vi "Reset Lock state.vi"(8 "error in (no error)":errorcluster, 9 "Boiler Simulation Controls":T1 {"Flame Sensor Value (%)" min=0.0 max=100.0 scale=0.0..100.0}, 10 "Indicator states in":T3 {"Time Count" format="%.2g"}, 11 "Runtime statuses in":T2) -> (0 "error out":errorcluster, 2 "Indicator states out":T3 {"Time Count" format="%.2g"}, 3 "Runtime statuses out":T2)   [LabVIEW 2014]
doc: "Checks runtime statuses and Control values. If Run Interlock is closed logs Boiler ready event and alows next state: Pre-Purge"
uses:
  Controls/Boiler Status Indicators.ctl
  Controls/Boiler runtime status indicators.ctl
  Controls/Boiler Simulation Controls.ctl
  Controls/Log file FGV action enum.ctl
  Controls/Log event enum.ctl
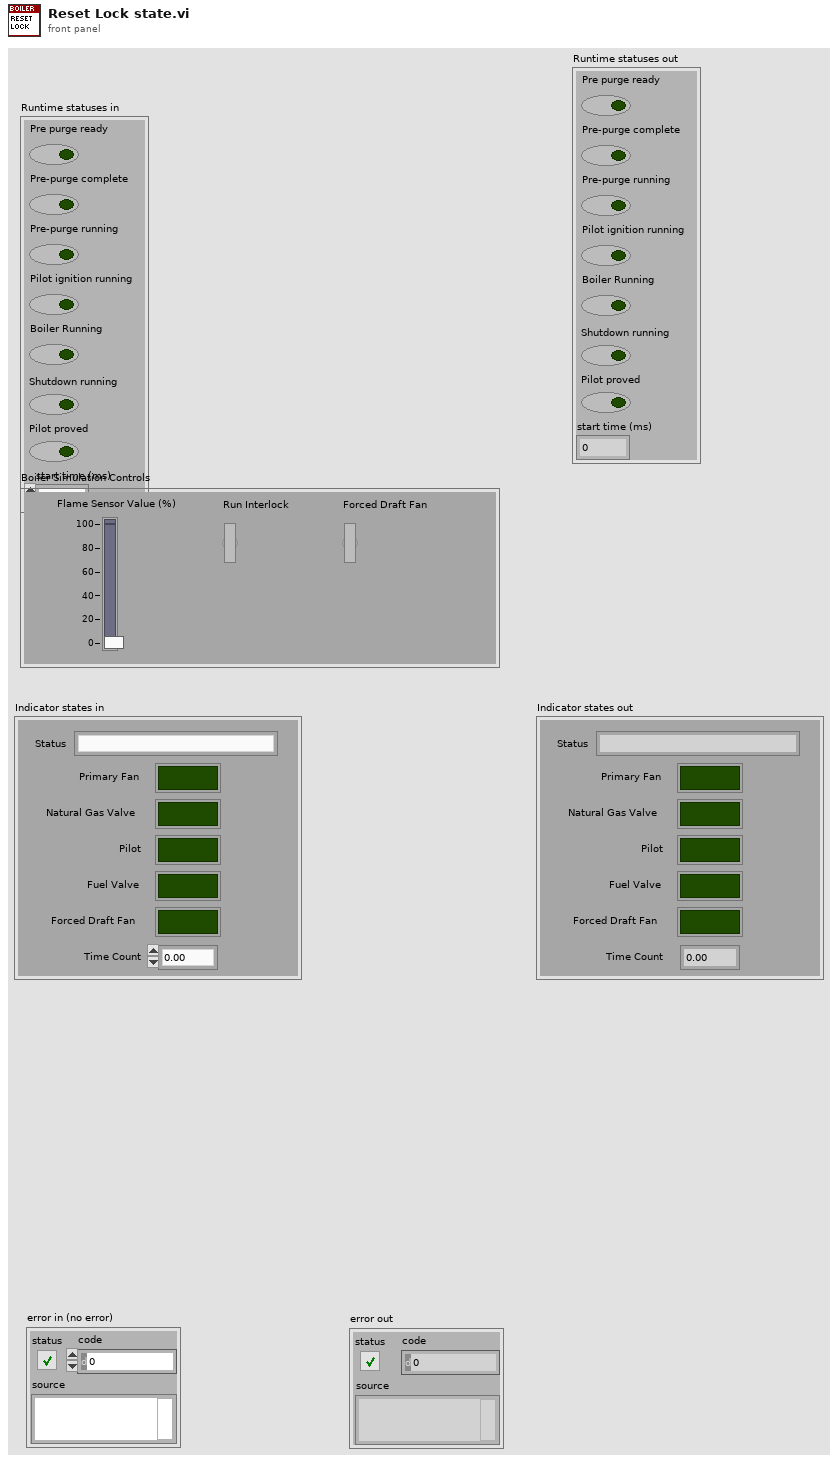
[diagram p1: front panel]
types:
  T1 = typedef "Boiler Simulation Controls.ctl" = cluster{"Flame Sensor Value (%)":dbl, "Run Interlock":bool, "Forced Draft Fan":bool}
  T2 = typedef "Boiler runtime status indicators.ctl" = cluster{"Pre purge ready":bool, "Pre-purge complete":bool, "Pre-purge running":bool, "Pilot ignition running":bool, "Boiler Running":bool, "Shutdown running":bool, "Pilot proved":bool, "start time (ms)":u32}
  T3 = typedef "Boiler Status Indicators.ctl" = cluster{"Status":string, "Primary Fan":bool, "Natural Gas Valve":bool, "Pilot":bool, "Fuel Valve":bool, "Forced Draft Fan":bool, "Time Count":dbl}
  T4 = typedef "Log event enum.ctl" = enum16{"Boiler Initialized", "Boiler Ready", "Start Pre-Purge", "Pre-Purge Complete", "Pilot ON", "Pilot proved", "Forced Draft Fan ON", "Boiler Running", "Start Shutdown Purge", "Shutdown Purge Complete"}
  T5 = typedef "Log file FGV action enum.ctl" = enum16{"open log file", "log event", "close log file"}
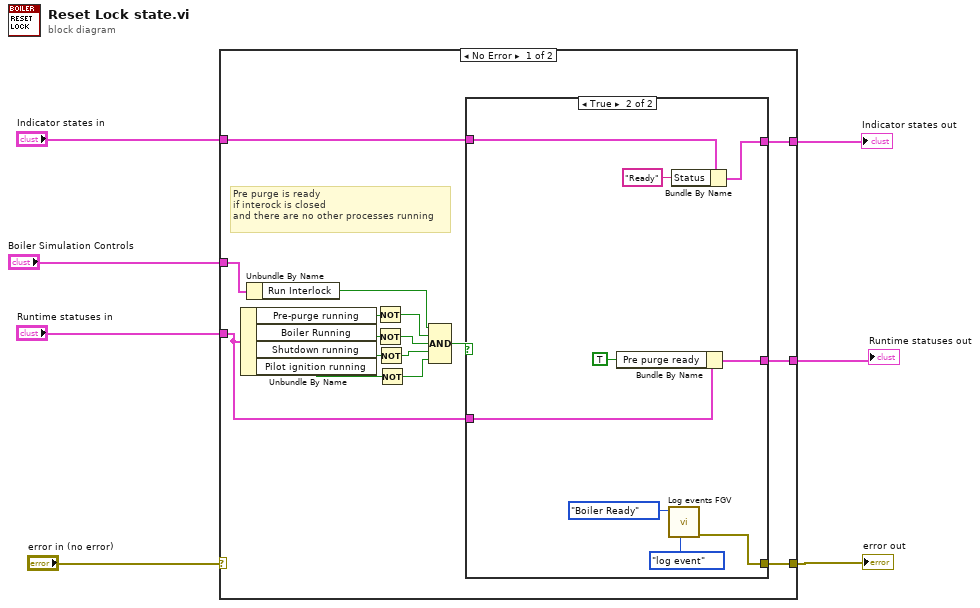
[diagram p0: block diagram]
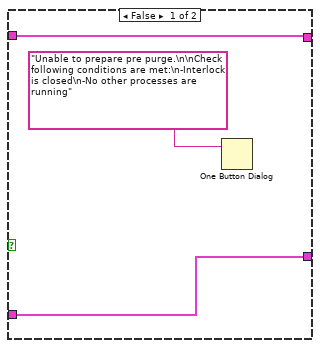
[diagram p2: hidden frame]
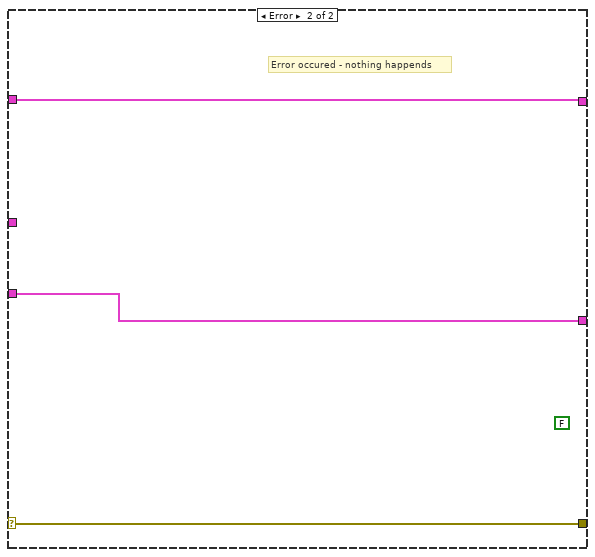
[diagram p3: hidden frame]
diagram:
  n1 = case shown="No Error" "error in (no error)" {
    selector: "error in (no error)" -> [_ w38]
    tunnel: [w8 w38] -> w6
    tunnel: "Runtime statuses in" -> [w12 w36]
    tunnel: "Boiler Simulation Controls" -> [w13 _]
    tunnel: "Indicator states in" -> [w16 w37]
    tunnel: [w15 w37] -> w2
    tunnel: [w11 w36] -> w1
    frame No Error {
      # "Pre purge is ready\nif interock is closed \nand there are no other processes running"
      n2 = Unbundle By Name(w12) -> ("Pre-purge running"=w23:bool, "Boiler Running"=w21:bool, "Shutdown running"=w22:bool, "Pilot ignition running"=w10:bool)
      n3 = Unbundle By Name(w13) -> ("Run Interlock"=w14:bool)
      n4 = Not(x=w23) -> (.not. x?=w20:bool)
      n5 = Not(x=w21) -> (.not. x?=w19:bool)
      n6 = Not(x=w22) -> (.not. x?=w18:bool)
      n7 = Not(x=w10) -> (.not. x?=w9:bool)
      n8 = Compound Arithmetic op=AND(w14, w20, w19, w18, w9) -> (w17:bool)
      n9 = case shown="True" w17 {
        tunnel: w16 -> [w26 w35]
        tunnel: [w26 w34] -> w15
        tunnel: w12 -> [w25 w32]
        tunnel: [w25 w31] -> w11
        tunnel: [_ w27] -> w8
        frame False {
          n10 = One Button Dialog(message="Unable to prepare pre purge.\n\nCheck following conditions are met:\n-Interlock is closed\n-No other processes are running") -> ()  [unwired: 1 in, 1 out]
        }
        frame True {
          n11 = Bundle By Name(cluster=w32, "Pre purge ready"=TRUE) -> (w31:T2)
          n12 = call "Log events FGV.vi"("action"=Log_file_FGV_action_enum."log event", "Log event"=Log_event_enum."Boiler Ready") -> ("error out"=w27:errorcluster)  [unwired: 9 in]
          n13 = Bundle By Name(cluster=w35, "Status"="Ready") -> (w34:T3)
        }
      }
    }
    frame Error {
      (unwired) FALSE
      # "Error occured - nothing happends"
    }
  }
  "Indicator states out" <- w2
  "error out" <- w6
  "Runtime statuses out" <- w1
